vi "Begin.vi"(8 "error in":errorcluster) -> (0 "error out":errorcluster)   [LabVIEW 2023]
doc: "Called before other user functions, this VI is expected to open initial I/O refnums, load in file data, and do all program initialization. Notice that the <B>error out</B> terminal is simply used for data flow. Wiring it to other structures or subVIs ensures that this VI runs first."
uses:
  <vilib>/Rock Robotics/WPI/DriverStation/WPI_DriverStationRobotMode2.ctl
  ctrl defs/ctrl pivot select.ctl
  Robot Global Data.vi
  <vilib>/Rock Robotics/Network Tables/NT Write String Array.vi
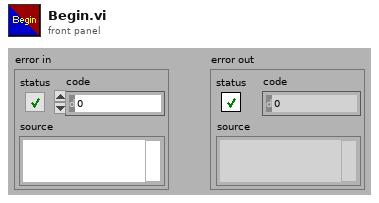
[diagram p1: front panel]
types:
  T1 = typedef "WPI_DriverStationRobotMode2.ctl" = enum16{"Autonomous Disabled", "Autonomous Enabled", "Teleop Disabled", "Teleop Enabled", "Disconnected", "Finish", "Test Disabled", "Test Enabled", "Emergency Stopped"}
  T2 = typedef "ctrl pivot select.ctl" = enum16{"geometric center", "CG", "FL", "FR", "RR", "RL", "other"}
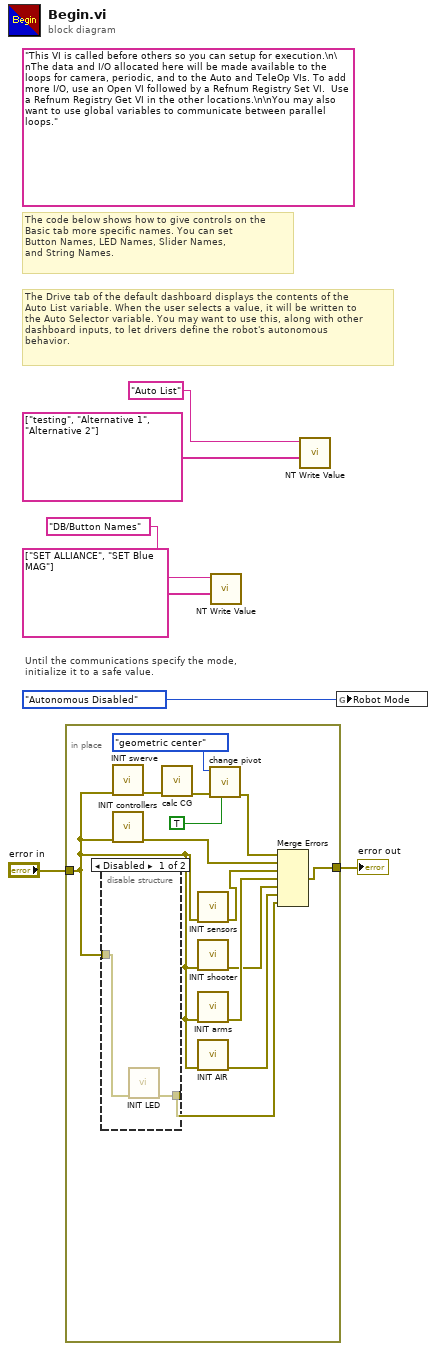
[diagram p0: block diagram]
diagram:
  (unwired) "This VI is called before others so you can setup for execution.\n\nThe data and I/O allocated here will be made available to the loops for camera, periodic, and to the Auto and TeleOp VIs. To add more I/O, use an Open VI followed by a Refnum Registry Set VI.  Use a Refnum Registry Get VI in the other locations.\n\nYou may also want to use global variables to communicate between parallel loops."
  # "The Drive tab of the default dashboard displays the contents of the\nAuto List variable. When the user selects a value, it will be written to\nthe Auto Selector variable. You may want to use this, along with other\ndashboard inputs, to let drivers define the robot's autonomous\nbehavior."
  # "The code below shows how to give controls on the\nBasic tab more specific names. You can set\nButton Names, LED Names, Slider Names,\nand String Names."
  # "Until the communications specify the mode,\ninitialize it to a safe value."
  n1 = in-place {
    in-place-border: "error in" -> [w13]
    in-place-border: [w15] -> w1
    n2 = disable-structure shown="Disabled" {
      disable-tunnel: w13 -> [w22 _]
      disable-tunnel: [w21 _] -> w14
      frame Disabled {
        n3 = call "INIT LED.vi"("error in (no error)"=w22) -> ("error out"=w21:errorcluster)  [unwired: 10 in]
      }
      frame Enabled {
      }
    }
    n4 = call "INIT swerve.vi"("error in (no error)"=w13) -> ("error out"=w20:errorcluster)  [unwired: 10 in]
    n5 = call "INIT controllers.vi"("error in (no error)"=w13) -> ("error out"=w16:errorcluster)  [unwired: 10 in]
    n6 = call "calc CG.vi"("error in (no error)"=w20) -> ("error out"=w19:errorcluster)  [unwired: 10 in]
    n7 = call "INIT sensors.vi"("error in (no error)"=w13) -> ("error out"=w9:errorcluster)  [unwired: 10 in]
    n8 = call "INIT shooter.vi"("error in (no error)"=w13) -> ("error out"=w10:errorcluster)  [unwired: 10 in]
    n9 = call "INIT arms.vi"("error in (no error)"=w13) -> ("error out"=w12:errorcluster)  [unwired: 10 in]
    n10 = call "INIT AIR.vi"("error in (no error)"=w13) -> ("error out"=w11:errorcluster)  [unwired: 10 in]
    n11 = call "change pivot.vi"("force recalc?"=TRUE, "error in (no error)"=w19, "select pivot point"=ctrl_pivot_select."geometric center") -> ("error out"=w17:errorcluster)  [unwired: 8 in]
    n12 = Merge Errors(w17, w16, w9, w12, w10, w11, w14) -> (w15:errorcluster)
  }
  "error out" <- w1
  n13 = call-poly <vilib>:"NT Write Value.vi"("value"=string[] ["SET ALLIANCE", "SET Blue MAG"], "name"="DB/Button Names" ("Name")) -> ()  [unwired: 9 in, 1 out]
  n14 = call-poly <vilib>:"NT Write Value.vi"("value"=string[] ["testing", "Alternative 1", "Alternative 2"] ("String Array"), "name"="Auto List" ("Name")) -> ()  [unwired: 9 in, 1 out]
  n15 = global write "Robot Global Data.vi" "Robot Mode"(WPI_DriverStationRobotMode2."Autonomous Disabled" ("Robot Mode")) -> ()
